vi "Write Image Path.vi"(8 "error in (no error)":errorcluster, 10 "Image Path":string, 11 "Save Image in":refnum<class "Save Image.lvclass">) -> (0 "error out":errorcluster, 3 "Save Image out":refnum<class "Save Image.lvclass">)   [LabVIEW 2018, in "Save Image.lvclass"]
uses:
  Save Image.lvclass
  Save Image.lvclass/Save Image.ctl
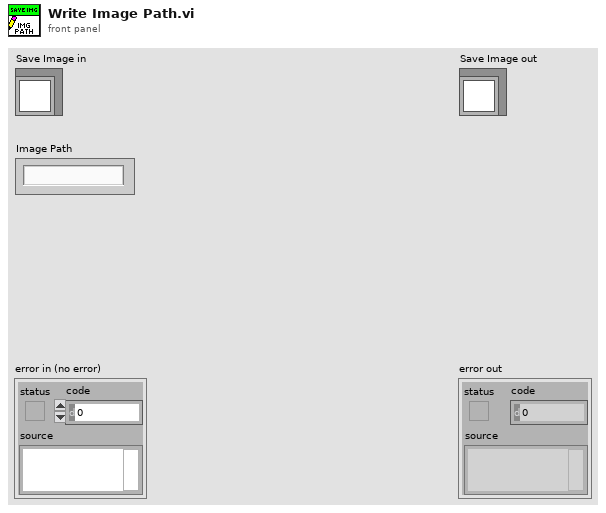
[diagram p1: front panel]
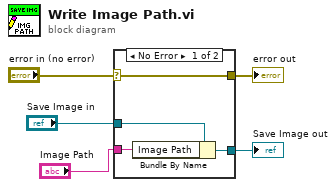
[diagram p0: block diagram]
diagram:
  n1 = case shown="No Error" "error in (no error)" {
    selector: "error in (no error)" -> [w7 w10]
    tunnel: [w7 w10] -> w4
    tunnel: [w9 w11] -> w2
    tunnel: "Save Image in" -> [w6 w11]
    tunnel: "Image Path" -> [w8 _]
    frame No Error {
      n2 = Bundle By Name(cluster=w6, "Image Path"=w8) -> (w9:refnum<class "Save Image.lvclass">)
    }
    frame Error {
    }
  }
  "error out" <- w4
  "Save Image out" <- w2
